vi "Custom Item Symbols-Set Symbol.vi"(8 "error in (no error)":errorcluster, 9 "Image":T1, 10 "Index":i32, 11 "TreeControl in":refnum<class "TreeControl.lvclass">) -> (0 "error out":errorcluster, 3 "TreeControl out":refnum<class "TreeControl.lvclass">)   [LabVIEW 2015, in "TreeControl.lvclass"]
doc: "Sets the image of an item symbol.\n\n If you want to use a picture to set the symbol, use the Picture to Pixmap VI to convert the data to an <b>image data</b> cluster before using this method. The <b>image</b> cluster you wire to this method is similar to the <b>image data</b> input of the Write JPEG File, Write PNG File, and Write BMP File VIs.\n\nQControl Class wrapper around the <b>TreeControl : Custom Item Symbols:Set To Custom Symbol Method</b>.\n<b> </b> <b> </b>\n©2016 Q Software Innovations, LLC (QSI)\nwritten by Quentin Alldredge\nproduced in LabVIEW 2015\n\nsupport@qsoftwareinnovations.com\nwww.qsoftwareinnovations.com\n\nAll rights reserved.\n\nRedistribution and use in source and binary forms, with or without modification, are permitted provided that the following conditions are met:\n\n * Redistributions of source code must retain the above copyright notice, this list of conditions and the following disclaimer.\n * Redistributions in binary form must reproduce the above copyright notice, this list of conditions and the following disclaimer in the documentation and/or other materials provided with the distribution.\n * Neither the name of Q Software Innovations, LLC. nor the names of its contributors may be used to endorse or promote products derived from this software without specific prior written permission.\n\nTHIS SOFTWARE IS PROVIDED BY THE COPYRIGHT HOLDERS AND CONTRIBUTORS \"AS IS\" AND ANY EXPRESS OR IMPLIED WARRANTIES, INCLUDING, BUT NOT LIMITED TO, THE IMPLIED WARRANTIES OF MERCHANTABILITY AND FITNESS FOR A PARTICULAR PURPOSE ARE DISCLAIMED. IN NO EVENT SHALL THE COPYRIGHT OWNER OR CONTRIBUTORS BE LIABLE FOR ANY DIRECT, INDIRECT, INCIDENTAL, SPECIAL, EXEMPLARY, OR CONSEQUENTIAL DAMAGES (INCLUDING, BUT NOT LIMITED TO, PROCUREMENT OF SUBSTITUTE GOODS OR SERVICES; LOSS OF USE, DATA, OR PROFITS; OR BUSINESS INTERRUPTION) HOWEVER CAUSED AND ON ANY THEORY OF LIABILITY, WHETHER IN CONTRACT, STRICT LIABILITY, OR TORT (INCLUDING NEGLIGENCE OR OTHERWISE) ARISING IN ANY WAY OUT OF THE USE OF THIS SOFTWARE, EVEN IF ADVISED OF THE POSSIBILITY OF SUCH DAMAGE."
uses:
  TreeControl.lvclass
  <vilib>/picture/picture.llb/imagedata.ctl
  TreeControl.lvclass/TreeControl.ctl
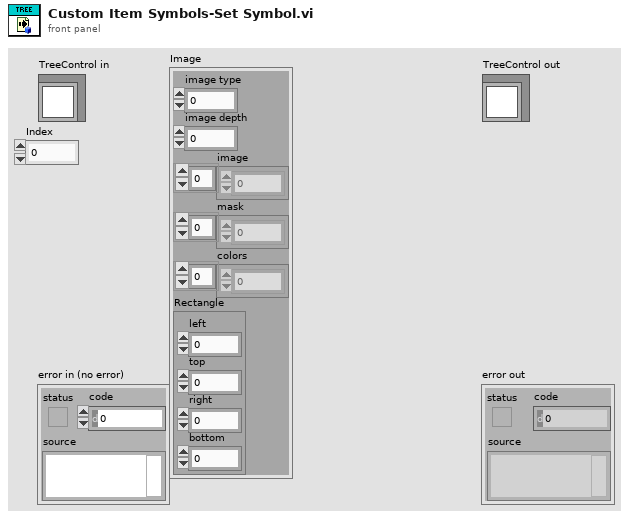
[diagram p1: front panel]
types:
  T1 = typedef "imagedata.ctl" = cluster{"image type":i32, "image depth":i32, "image":u8[], "mask":u8[], "colors":u32[], "Rectangle":cluster{"left":i16, "top":i16, "right":i16, "bottom":i16}}
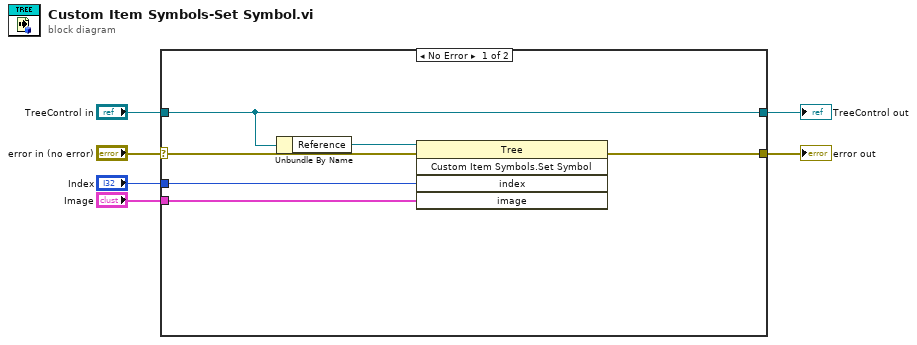
[diagram p0: block diagram]
diagram:
  n1 = case shown="No Error" "error in (no error)" {
    selector: "error in (no error)" -> [w12 w14]
    tunnel: [w11 w14] -> w5
    tunnel: [w10 w13] -> w3
    tunnel: "TreeControl in" -> [w10 w13]
    tunnel: "Index" -> [w8 _]
    tunnel: "Image" -> [w7 _]
    frame No Error {
      n2 = Unbundle By Name(w10) -> ("Reference"=w9:refnum<vi>)
      n3 = invoke class="Tree" method="Custom Item Symbols.Set Symbol"(reference=w9, error in=w12, "index"=w8, "image"=w7) -> (error out=w11:errorcluster)  [unwired: 1 in, 4 out]
    }
    frame Error {
    }
  }
  "error out" <- w5
  "TreeControl out" <- w3
